vi "RELAX.vi"   [LabVIEW 2020]
uses:
  OP500/VG/VG_progressBar.vi
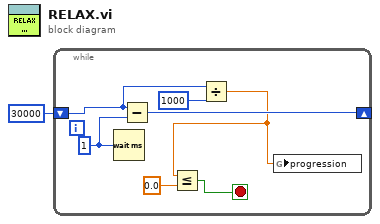
[diagram p0: block diagram]
diagram:
  n1 = while {
    shift-right: [w5] -> _
    shift-left: u32 30000 -> [w7]
    stop <- w4 stop-if-true
    w8 = u32 1 ("attente (ms)")
    n2 = Wait (ms)(milliseconds to wait=w8) -> ()  [unwired: 1 out]
    n3 = Subtract(x=w7, y=w8) -> (x-y=w5:u32)
    n4 = Divide(x=w7, y=u32 1000) -> (x/y=w3:dbl)
    n5 = Less Or Equal?(x=w3, y=0.0) -> (x <= y?=w4:bool)
    n6 = global write "VG_progressBar.vi" "progression"(w3) -> ()
  }
